vi "ImplementInterfaces.vi"(0 "ClassWriterNative":refnum<class "ClassWriter.lvclass">, 1 "ClassItemRefIn":refnum<vi>, 2 "InterfacesToImplement":T1, 5 "error in (no error)":errorcluster) -> (14 "ClassWriterNative":refnum<class "ClassWriter.lvclass">, 15 "ClassItemRefOut":refnum<vi>, 17 "Cancelled":bool, 19 "error out":errorcluster)   [LabVIEW 2020, in "ClassWriter.lvclass"]
uses:
  <resource>/Framework/Providers/Open_GDS/ClassProviders/Provider_BaseClassInterface/ClassWriter_class/ClassWriter.lvclass
  <resource>/Framework/Providers/Open_GDS/ClassProviders/Provider_BaseClassInterface/ClassWriter_class/InterfacesToImplement.ctl
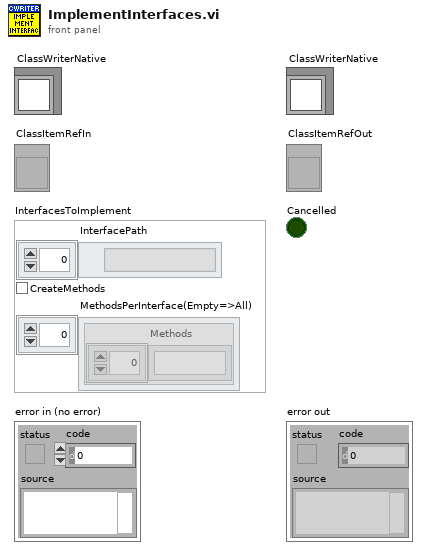
[diagram p1: front panel]
types:
  T1 = typedef "ClassWriter.lvclass/InterfacesToImplement.ctl" = cluster{"InterfacePath":path[], "CreateMethods":bool, "MethodsPerInterface(Empty=>All)":cluster{"Methods":string[]}[]}
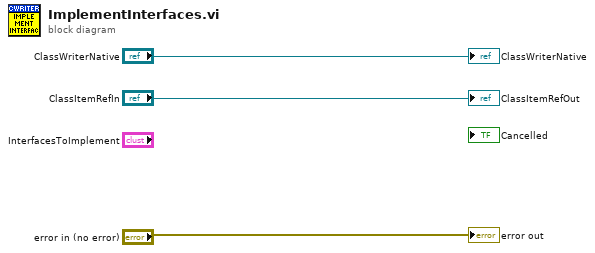
[diagram p0: block diagram]
diagram:
  "ClassWriterNative" <- "ClassWriterNative"
  "error out" <- "error in (no error)"
  "ClassItemRefOut" <- "ClassItemRefIn"
